vi "gen_sub_environment.vi"(11 "Environment in":T1) -> (3 "Environment out":T1)   [LabVIEW 2021]
uses:
  Environment.ctl
  Expression.ctl
  ExpressionType.ctl
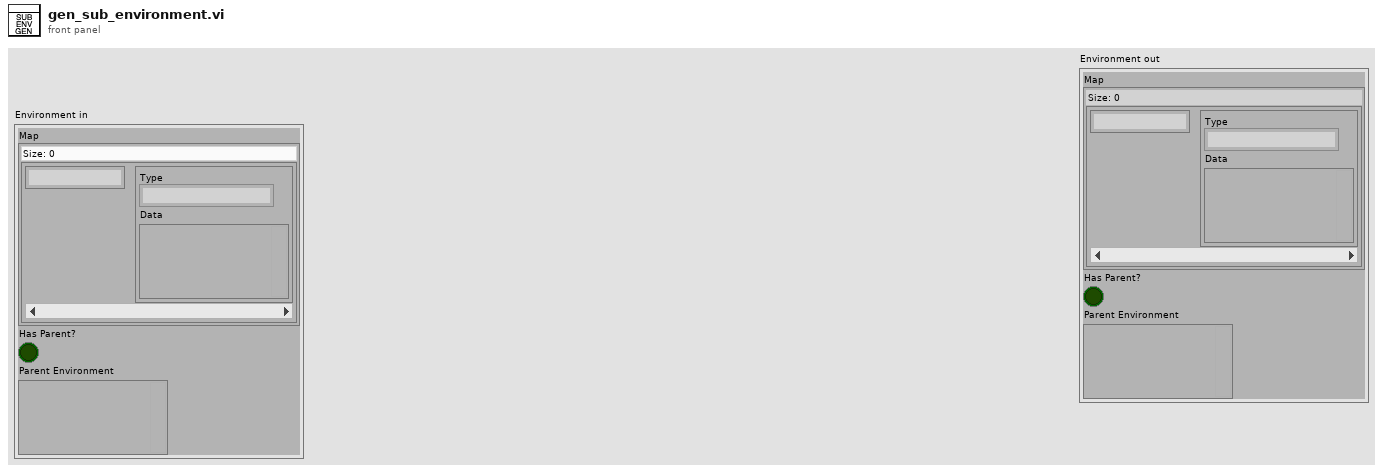
[diagram p1: front panel]
types:
  T1 = typedef "Environment.ctl" = cluster{"Map":map{string, T2}, "Has Parent?":bool, "Parent Environment":variant}
  T2 = typedef "Expression.ctl" = cluster{"Type":T3, "Data":variant}
  T3 = typedef "ExpressionType.ctl" = enum16{"number", "string", "symbol", "primitive", "list", "closure", "macro", "nil", "error"}
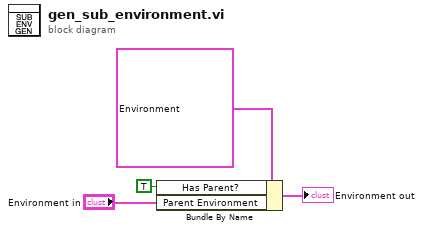
[diagram p0: block diagram]
diagram:
  n1 = Bundle By Name(cluster=T1 {"Map"={}, "Has Parent?"=FALSE, "Parent Environment"=variant} ("Environment in"), "Has Parent?"=TRUE, "Parent Environment"="Environment in") -> (→"Environment out":T1)
